vi "getArgumentInfoList.vi"(8 "error in (no error)":errorcluster, 11 "IList in":refnum<class "IList.lvclass">) -> (0 "error out":errorcluster, 2 "baseObjects out":refnum<class "IArgumentInfo.lvclass">[](array[class]))   [LabVIEW 2022 SP3, in "openDAQ.lvlib" / "daqCoreTypes.lvlib" / "IList.lvclass"]
uses:
  IList.lvclass
  IArgumentInfo/IArgumentInfo.lvclass
  Errors/TypeDef/errorCodes.ctl
  Errors/Errors.lvclass
  IIterator/IIterator.lvclass
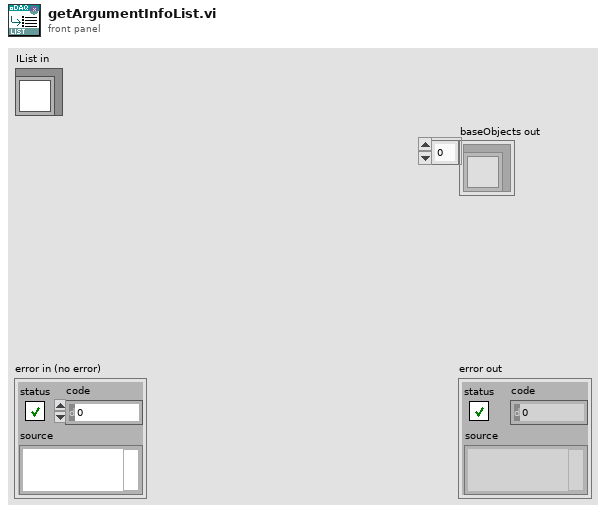
[diagram p1: front panel]
types:
  T1 = typedef "openDAQ.lvlib/daqCoreTypes.lvlib/Errors.lvclass/errorCodes.ctl" = u16
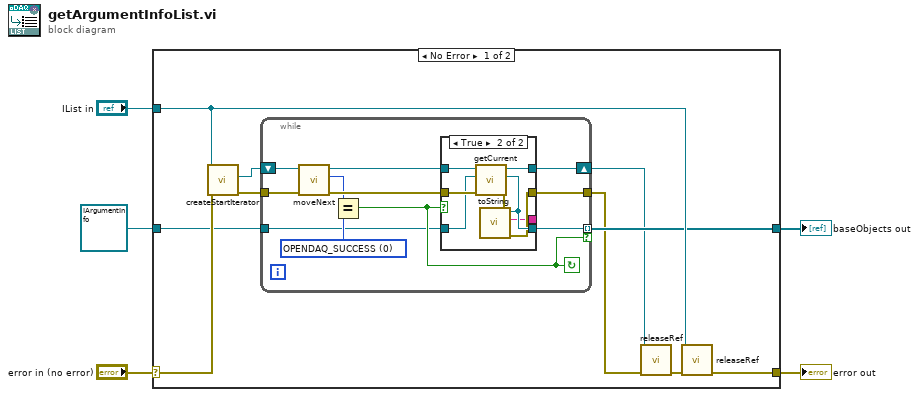
[diagram p0: block diagram]
diagram:
  n1 = case shown="No Error" "error in (no error)" {
    selector: "error in (no error)" -> [w11 w37]
    tunnel: [w15 w37] -> w4
    tunnel: "IList in" -> [w12 _]
    tunnel: refnum<class "IArgumentInfo.lvclass"> refnum ("openDAQ.lvlib:IBaseObject.lvlib:IArgumentInfo.lvlib:IArgumentInfo.lvclass") -> [w6 _]
    tunnel: [w10 _] -> w2
    frame No Error {
      n2 = call "createStartIterator.vi"("error in (no error)"=w11, "IList in"=w12) -> ("error out"=w13:errorcluster, "IIterator out"=w14:refnum<class "IIterator.lvclass">)  [unwired: 7 in, 1 out]
      n3 = while {
        tunnel: w13 -> [w24]
        tunnel: [w21] -> w8
        shift-right: [w20] -> w7
        shift-left: w14 -> [w25]
        tunnel: [w17] -> w10 mode=indexing if=w19
        tunnel: w6 -> [w16]
        stop <- w19 continue-if-true
        w18 = T1 0 items=["OPENDAQ_SUCCESS"=0, "OPENDAQ_NO_MORE_ITEMS"=5] ("errorCodes")
        n4 = call "moveNext.vi"("error in (no error)"=w24, "IIterator in"=w25) -> ("error out"=w26:errorcluster, "errorCode out"=w23:T1, "IIterator out"=w22:refnum<class "IIterator.lvclass">)  [unwired: 7 in]
        n5 = Equal?(x=w23, y=w18) -> (x = y?=w19:bool)
        n6 = case shown="True" w19 {
          tunnel: w22 -> [w27 w35]
          tunnel: w26 -> [w28 w36]
          tunnel: [w28 w30] -> w21
          tunnel: [w27 w34] -> w20
          tunnel: [_ w32] -> w17
          tunnel: w16 -> [_ w33]
          tunnel: [_ w29] -> _
          frame False {
          }
          frame True {
            n7 = call "getCurrent.vi"("error in (no error)"=w36, "baseObject in"=w33, "IIterator in"=w35) -> ("error out"=w31:errorcluster, "baseObject out"=w32:refnum<class "IArgumentInfo.lvclass">, "IIterator out"=w34:refnum<class "IIterator.lvclass">)  [unwired: 6 in]
            n8 = call-dynamic "toString.vi"("error in (no error)"=w31, "IBaseObject in"=w32) -> ("error out"=w30:errorcluster, "string"=w29:string)  [unwired: 7 in, 1 out]
          }
        }
      }
      n9 = call-dynamic "releaseRef.vi"("error in (no error)"=w8, "IBaseObject in"=w7) -> ("error out"=w9:errorcluster)  [unwired: 9 in]
      n10 = call-dynamic "releaseRef.vi"("error in (no error)"=w9, "IBaseObject in"=w12) -> ("error out"=w15:errorcluster)  [unwired: 9 in]
    }
    frame Error {
    }
  }
  "error out" <- w4
  "baseObjects out" <- w2
